vi "Value - Deprecated.vi"(11 "Value in":refnum<class "Value.lvclass">) -> ()   [LabVIEW 2020, in "Promises.lvlib" / "Value.lvclass"]
uses:
  Value.lvclass
panel:
  # "This VI is here to break children classes. This class/interface is no longer necessary to use the Promises library and should be removed as a parent of any classes."
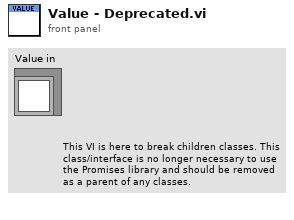
[diagram p1: front panel]
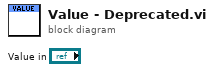
[diagram p0: block diagram]
diagram:
